vi "Path as Path (LabVIEW Path).vi"(9 "Path":path) -> (1 "Path":path)   [LabVIEW 2020, in "G-Unicode.lvlib"]
doc: "Converts the input path to a raw UTF-8 encoded LabVIEW path. Valid inputs are a UTF-8 Path class or LabVIEW path."
uses:
  Types/UTF-8 Path/UTF-8 Path.lvclass/UTF-8 Path.ctl
  G-Unicode.lvlib
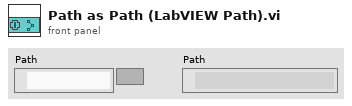
[diagram p1: front panel]
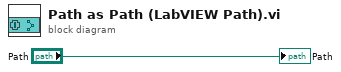
[diagram p0: block diagram]
diagram:
  "Path" <- "Path"
